vi "get FTR.vi"(8 "error in (no error)":errorcluster, 11 "Thorcam in":refnum<class "Thorcam.lvclass">) -> (0 "error out":errorcluster, 3 "Thorcam out":refnum<class "Thorcam.lvclass">)   [LabVIEW 2012, in "Thorcam.lvclass"]
uses:
  Thorcam.lvclass
  Thorcam.lvclass/Thorcam.ctl
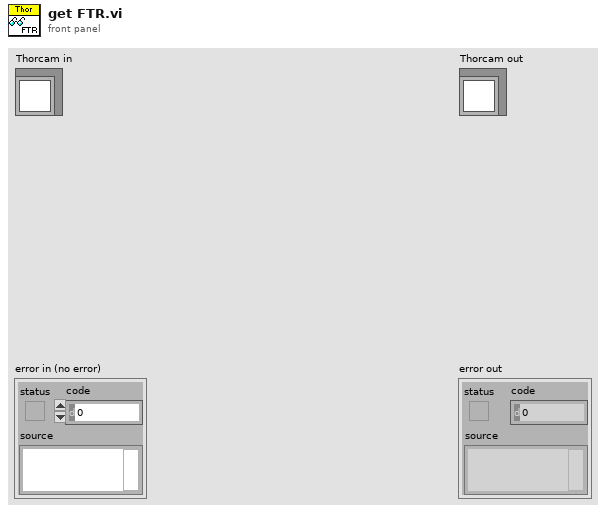
[diagram p1: front panel]
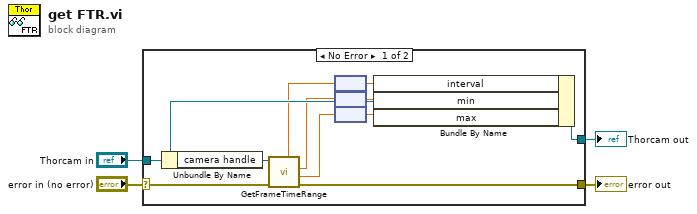
[diagram p0: block diagram]
diagram:
  n1 = case shown="No Error" "error in (no error)" {
    selector: "error in (no error)" -> [w14 w17]
    tunnel: [w13 w17] -> w3
    tunnel: [w11 w16] -> w1
    tunnel: "Thorcam in" -> [w12 w16]
    frame No Error {
      n2 = Unbundle By Name(w12) -> ("camera handle"=w15:u32)
      n3 = call <instrlib>:"GetFrameTimeRange.vi"("error in"=w14, "Camera Handle In"=w15) -> ("error out"=w13:errorcluster, "max"=w5:dbl, "min"=w6:dbl, "interval"=w10:dbl)  [unwired: 5 in, 1 out]
      n4 = node(w10) -> (w9:dbl[unit])
      n5 = node(w6) -> (w8:dbl[unit])
      n6 = node(w5) -> (w7:dbl[unit])
      n7 = Bundle By Name(cluster=w12, "interval"=w9, "min"=w8, "max"=w7) -> (w11:refnum<class "Thorcam.lvclass">)
    }
    frame Error {
    }
  }
  "error out" <- w3
  "Thorcam out" <- w1
